vi "Actor Destroy.vi"(11 "Dev Actor in":refnum<class "Dev Actor.lvclass">) -> (3 "Dev Actor out":refnum<class "Dev Actor.lvclass">)   [LabVIEW 2021, in "Dev Actor.lvlib" / "Dev Actor.lvclass"]
uses:
  Dev Actor.lvclass
  Dev Actor.lvclass/Dev Actor.ctl
  <vilib>/jettl/jettl/Actor/Actor/Actor.lvclass
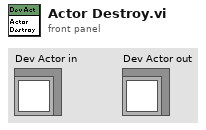
[diagram p1: front panel]
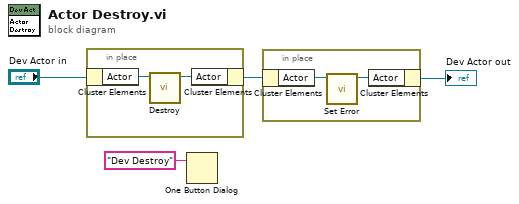
[diagram p0: block diagram]
diagram:
  n1 = in-place {
    n2 = in-place-cluster #1("Dev Actor in") -> ("Actor"=w5:refnum<class "Actor.lvclass">)
    n3 = call-dynamic "Destroy.vi"("Destroy in"=w5) -> ("Destroy out"=w6:refnum<class "Actor.lvclass">)  [unwired: 10 in]
    n4 = in-place-cluster #1("Actor"=w6) -> (w1:refnum<class "Dev Actor.lvclass">)
  }
  n5 = One Button Dialog(message="Dev Destroy") -> ()  [unwired: 1 in, 1 out]
  n6 = in-place {
    n7 = in-place-cluster #2(w1) -> ("Actor"=w8:refnum<class "Actor.lvclass">)
    n8 = call-dynamic "Set Error.vi"("Set Error in"=w8) -> ("Set Error out"=w7:refnum<class "Actor.lvclass">)  [unwired: 10 in]
    n9 = in-place-cluster #2("Actor"=w7) -> (→"Dev Actor out":refnum<class "Dev Actor.lvclass">)
  }
